vi "STOR.vi"(8 "error in (no error)":errorcluster, 9 "Local FilePath":path, 10 "Remote FileName":string, 11 "FTP in":refnum<class "FTP.lvclass">) -> (0 "error out":errorcluster, 3 "FTP out":refnum<class "FTP.lvclass">)   [LabVIEW 2020, in "FTP.lvlib" / "FTP.lvclass"]
uses:
  FTP.lvclass
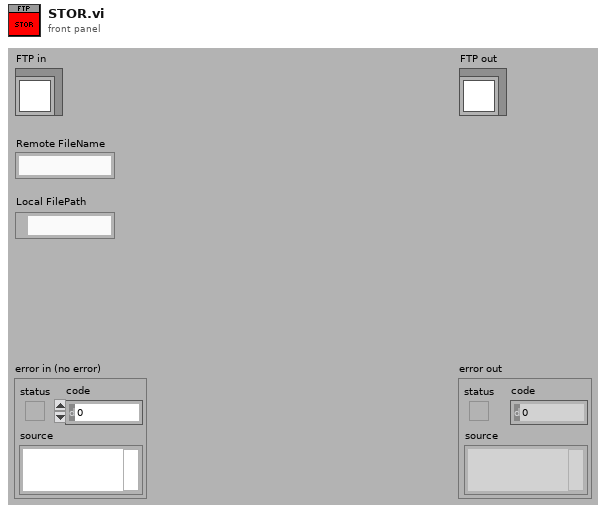
[diagram p1: front panel]
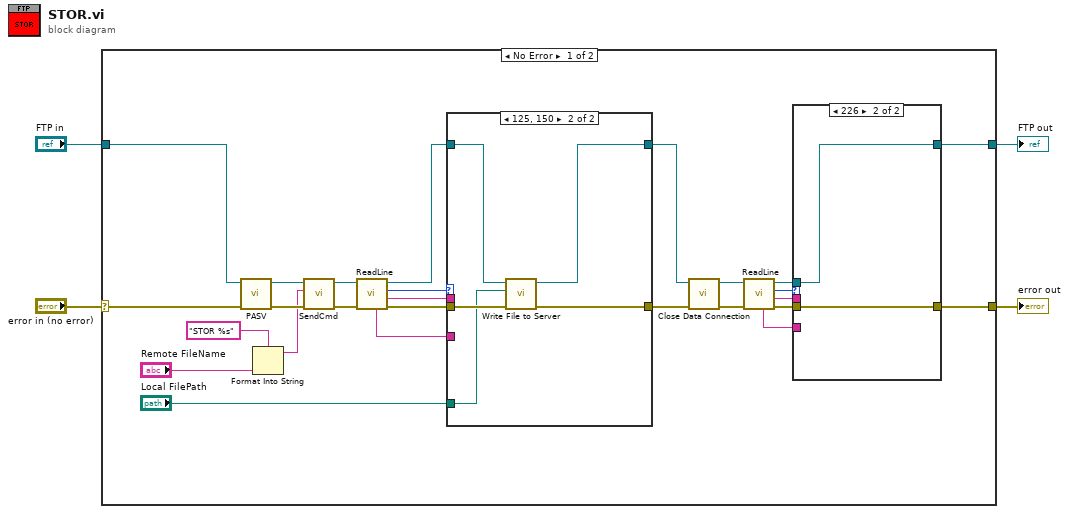
[diagram p0: block diagram]
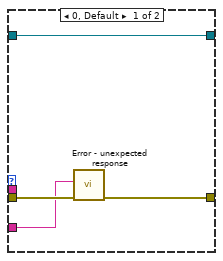
[diagram p2: hidden frame]
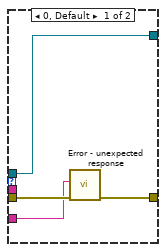
[diagram p3: hidden frame]
diagram:
  n1 = case shown="No Error" "error in (no error)" {
    selector: "error in (no error)" -> [w24 w47]
    tunnel: [w23 w47] -> w2
    tunnel: [w22 w46] -> w1
    tunnel: "FTP in" -> [w21 w46]
    frame No Error {
      n2 = call "PASV.vi"("error in (no error)"=w24, "FTP in"=w21) -> ("error out"=w27:errorcluster, "FTP out"=w28:refnum<class "FTP.lvclass">)  [unwired: 8 in]
      n3 = Format Into String(format string="STOR %s" ("cmd"), "Remote FileName") -> (resulting string=w18:string)  [unwired: 2 in, 1 out]
      n4 = call "SendCmd.vi"("error in (no error)"=w27, "cmd"=w18, "FTP in"=w28) -> ("error out"=w29:errorcluster, "FTP out"=w30:refnum<class "FTP.lvclass">)  [unwired: 7 in]
      n5 = call "ReadLine.vi"("error in (no error)"=w29, "FTP in"=w30) -> ("error out"=w26:errorcluster, "Line"=w8:string, "code"=w9:i32, "FTP out"=w25:refnum<class "FTP.lvclass">, "Full Line"=w6:string)  [unwired: 5 in]
      n6 = case shown="125, 150" w9 {
        tunnel: w26 -> [w33 w39]
        tunnel: w25 -> [w34 w37]
        tunnel: [w31 w38] -> w11
        tunnel: [w34 w36] -> w10
        tunnel: w8 -> [_ _]
        tunnel: "Local FilePath" -> [_ w35]
        tunnel: w6 -> [w32 _]
        frame 0, Default {
          n7 = call "Error - unexpected response.vi"("error in (no error)"=w33, "Full Response"=w32) -> ("error out"=w31:errorcluster)  [unwired: 9 in]
        }
        frame 125, 150 {
          n8 = call "Write File to Server.vi"("error in (no error)"=w39, "Local FilePath"=w35, "FTP in"=w37) -> ("error out"=w38:errorcluster, "FTP out"=w36:refnum<class "FTP.lvclass">)  [unwired: 7 in]
        }
      }
      n9 = call "Close Data Connection.vi"("error in (no error)"=w11, "FTP in"=w10) -> ("error out"=w17:errorcluster, "FTP out"=w16:refnum<class "FTP.lvclass">)  [unwired: 8 in]
      n10 = call "ReadLine.vi"("error in (no error)"=w17, "FTP in"=w16) -> ("error out"=w15:errorcluster, "Line"=w12:string, "code"=w14:i32, "FTP out"=w13:refnum<class "FTP.lvclass">, "Full Line"=w5:string)  [unwired: 5 in]
      n11 = case shown="226" w14 {
        tunnel: w15 -> [w42 w44]
        tunnel: [w40 w44] -> w23
        tunnel: w13 -> [w43 w45]
        tunnel: [w43 w45] -> w22
        tunnel: w12 -> [_ _]
        tunnel: w5 -> [w41 _]
        frame 0, Default {
          n12 = call "Error - unexpected response.vi"("error in (no error)"=w42, "Full Response"=w41) -> ("error out"=w40:errorcluster)  [unwired: 9 in]
        }
        frame 226 {
        }
      }
    }
    frame Error {
    }
  }
  "error out" <- w2
  "FTP out" <- w1
